vi "IPFPDBL.vi"(3 "Number":dbl) -> (0 "Fractional part":dbl, 1 "Integer part":dbl)   [LabVIEW 2017, in "GPNumeric.lvlib"]
doc: "Splits floating point <B>Number</B> into <B>Integer part</B> and <B>Fractional part</B>.\n\nThis VI is inlined.\n\nSteen Schmidt\nGPower\n16/5 2014"
uses:
  GPNumeric.lvlib
panel:
  # "Copyright © 2014\nGPower\nSee enclosed license file for terms and conditions"
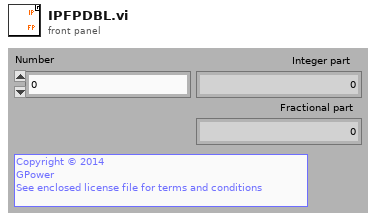
[diagram p1: front panel]
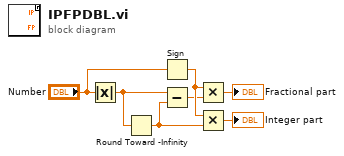
[diagram p0: block diagram]
diagram:
  n1 = Absolute Value(x="Number") -> (abs(x)=w3:dbl)
  n2 = Round Toward -Infinity(1:w3) -> (0:w2:dbl)
  n3 = Sign(1:"Number") -> (0:w4:dbl)
  n4 = Subtract(x=w3, y=w2) -> (x-y=w1:dbl)
  n5 = Multiply(x=w4, y=w1) -> (x*y=→"Fractional part":dbl)
  n6 = Multiply(x=w4, y=w2) -> (x*y=→"Integer part":dbl)
